vi "WS1050 OFFSET CAL.vi"(8 "error in":errorcluster, 10 "OFFSET CAL":bool=TRUE) -> (0 "error out":errorcluster, 3 "AD7747 Values":string[][](table))   [LabVIEW 2012]
uses:
  WS_VCAP Driver 029/Source/WSVCAP Shell/Type Defs/WSVCAP SHL I2C DUT Mask Mode Enum.ctl
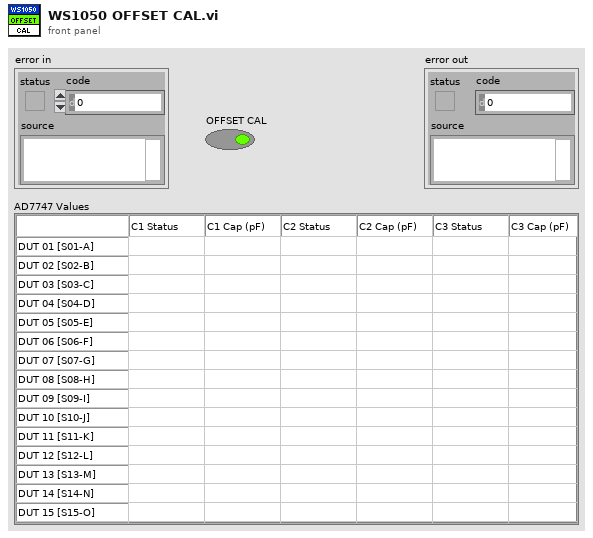
[diagram p1: front panel]
types:
  T1 = typedef "WSVCAP SHL I2C DUT Mask Mode Enum.ctl" = enum16{"Custom", "C1", "C2", "C3", "All"}
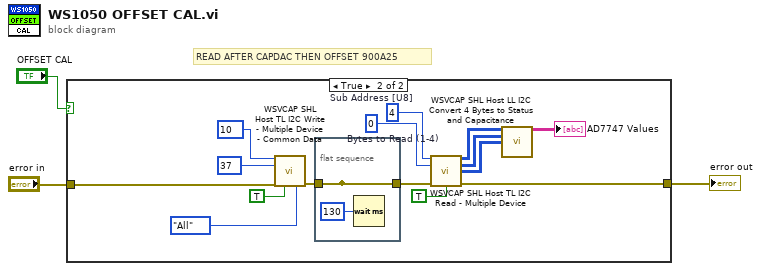
[diagram p0: block diagram]
diagram:
  # "READ AFTER CAPDAC THEN OFFSET 900A25"
  n1 = case shown="True" "OFFSET CAL" {
    tunnel: "error in" -> [w4 w19]
    tunnel: [w4 w10] -> w3
    frame False {
    }
    frame True {
      w16 = u8 4  # Bytes to Read (1-4)
      w17 = u8 0  # Sub Address [U8]
      n2 = call "WSVCAP SHL Host TL I2C Write - Multiple Device - Common Data.vi"("Sub Address"=u8 10, "Data Out [U8]"=u8 37 ("Sub Address"), "error in"=w19, "Log (T)"=TRUE, "DUT Mask Mode (All)"=WSVCAP_SHL_I2C_DUT_Mask_Mode_Enum."All") -> ("error out"=w18:errorcluster)  [unwired: 10 in]
      n3 = flat-sequence {
        tunnel: w18 -> [w20]
        tunnel: [w20] -> _
        tunnel: [w20] -> w11
        frame #0 {
          n4 = Wait (ms)(milliseconds to wait=u32 130) -> ()  [unwired: 1 out]
        }
      }
      n5 = call "WSVCAP SHL Host TL I2C Read - Multiple Device.vi"("Bytes to Read (1-4)"=w16, "Sub Address [U8]"=w17, "error in"=w11, "Log (T)"=TRUE) -> ("C1:1-36 Read Data [U8]"=w15:u8[][], "C2:1-36 Read Data [U8]"=w14:u8[][], "C3:1-36 Read Data [U8]"=w12:u8[][], "error out"=w10:errorcluster)  [unwired: 8 in]
      n6 = call "WSVCAP SHL Host LL I2C Convert 4 Bytes to Status and Capacitance.vi"("C1:1-36 Read Data [U8]"=w15, "C2_1-36 Read Data [U8]"=w14, "C3_1-36 Read Data [U8]"=w12) -> ("AD7747 Values"=→"AD7747 Values":string[][])  [unwired: 12 in]
    }
  }
  "error out" <- w3
